vi "Solve2.vi"(8 "Error In":errorcluster, 11 "object in":refnum<class "2024_5.lvclass">) -> (0 "Error Out":errorcluster, 2 "Result":u64, 3 "object out":refnum<class "2024_5.lvclass">)   [LabVIEW 2023, in "2024_5.lvclass"]
uses:
  2024_5.lvclass
  2024_5.lvclass/2024_5.ctl
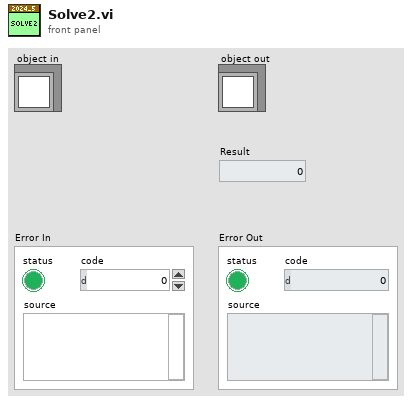
[diagram p1: front panel]
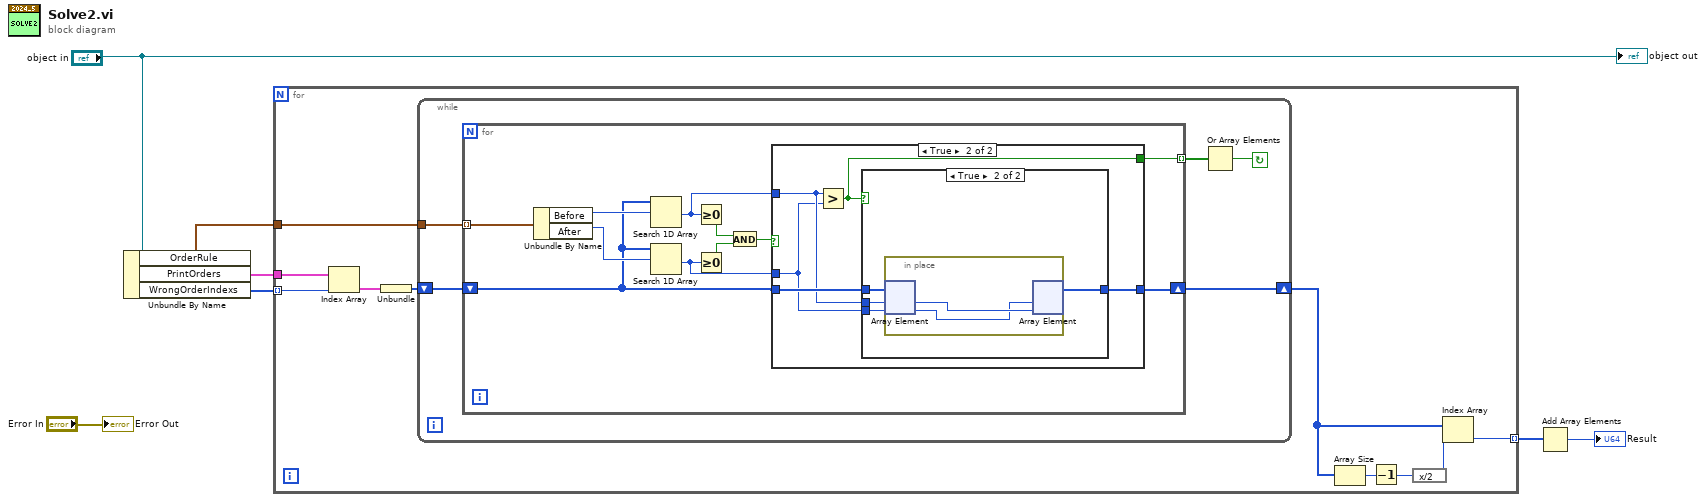
[diagram p0: block diagram]
diagram:
  n1 = Unbundle By Name("object in") -> ("OrderRule"=w3:cluster{"Before":i64, "After":i64}[], "PrintOrders"=w5:cluster{"Pages":i32[]}[], "WrongOrderIndexs"=w4:i32[])
  n2 = for {
    tunnel: w5 -> [w17]
    tunnel: w4 -> [w16] mode=indexing
    tunnel: w3 -> [w14]
    tunnel: [w8] -> w2 mode=indexing
    n3 = Index Array(array=w17, index=w16) -> (element=w15:cluster{"Pages":i32[]})
    n4 = Unbundle(w15) -> ("Pages"=w13:i32[])
    n5 = while {
      tunnel: w14 -> [w22]
      shift-right: [w20] -> w9
      shift-left: w13 -> [w21]
      stop <- w18 continue-if-true
      n6 = for {
        tunnel: w22 -> [w29] mode=indexing
        shift-right: [w26] -> w20
        shift-left: w21 -> [w27]
        tunnel: [w23] -> w19 mode=indexing
        n7 = Unbundle By Name(w29) -> ("Before"=w33:i64, "After"=w32:i64)
        n8 = Search 1D Array(1D array=w27, element=w33) -> (index of element=w25:i32)  [unwired: 1 in]
        n9 = Search 1D Array(1D array=w27, element=w32) -> (index of element=w24:i32)  [unwired: 1 in]
        n10 = Greater Or Equal To 0?(x=w25) -> (x >= 0?=w30:bool)
        n11 = Greater Or Equal To 0?(x=w24) -> (x >= 0?=w31:bool)
        n12 = And(x=w30, y=w31) -> (x .and. y?=w28:bool)
        n13 = case shown="True" w28 {
          tunnel: w27 -> [w34 w39]
          tunnel: [w34 w38] -> w26
          tunnel: w25 -> [_ w37]
          tunnel: w24 -> [_ w36]
          tunnel: [_ w35] -> w23
          frame False {
          }
          frame True {
            n14 = Greater?(x=w37, y=w36) -> (0:w35:bool)
            n15 = case shown="True" w35 {
              tunnel: w39 -> [w40 w44]
              tunnel: [w40 w43] -> w38
              tunnel: w37 -> [_ w42]
              tunnel: w36 -> [_ w41]
              frame False {
              }
              frame True {
                n16 = in-place {
                  n17 = in-place-array #1(w44, w42, w41) -> (w46:i32, w45:i32)
                  n18 = in-place-array #1(w45, w46) -> (w43:i32[])  [unwired: 2 out]
                }
              }
            }
          }
        }
      }
      n19 = Or Array Elements(Boolean array=w19) -> (logical OR=w18:bool)
    }
    n20 = Array Size(array=w9) -> (size(s)=w12:i32)
    n21 = Decrement(x=w12) -> (x-1=w11:i32)
    n22 = expression code="x/2"(w11) -> (w10:i32)
    n23 = Index Array(array=w9, index=w10) -> (element=w8:i32)
  }
  n24 = Add Array Elements(numeric array=w2) -> (sum=→"Result":i32)
  "Error Out" <- "Error In"
  "object out" <- "object in"
